vi "Keithley DMM7510 Acquire Triggered Multiple.vi"() -> ()   [LabVIEW 2015]
doc: "This example shows how to configure a measurement, set up triggering, trigger a measurement, and retrieve a measurement. It shows how to use the low-level Data VIs to retrieve data from the DMM."
uses:
  Keithley DMM7510.lvlib
panel:
  in  "Function":u16(ring) items=["Voltage: DC", "Voltage: AC", "Current: DC", "Current: AC", "2W Resistance", "4W Resistance", "Diode", "Capacitance", "Temperature", "Continuity", "Frequency", "Period", "Ratio"]
  in  "Sample Count (10)":i32=10 format="%#.6g"
  in  "Timeout (10000 ms)":i32=10000 format="%#.6g"
  out "Waveform Chart":dbl[](graph)
  in  "VISA resource name":refnum<visa-resource-name>
  # "(c) 2015 Keithley Instruments,,  ALL RIGHTS RESERVED."
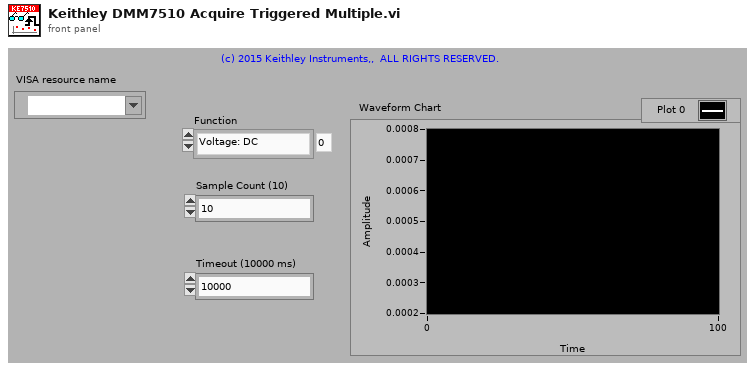
[diagram p1: front panel]
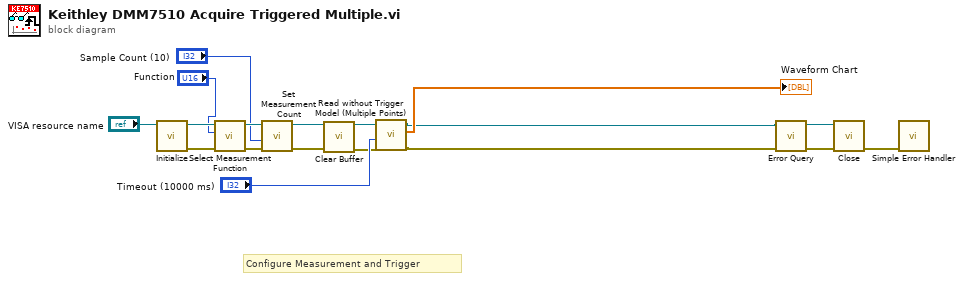
[diagram p0: block diagram]
diagram:
  # "Configure Measurement and Trigger"
  n1 = call "Initialize.vi"("VISA resource name"="VISA resource name") -> ("error out"=w14:errorcluster, "VISA resource name out"=w13:refnum<visa-resource-name>)  [unwired: 9 in]
  n2 = call "Select Measurement Function.vi"("error in (no error)"=w14, "Function"="Function", "VISA resource name"=w13) -> ("error out"=w11:errorcluster, "VISA resource name out"=w10:refnum<visa-resource-name>)  [unwired: 7 in]
  n3 = call "Set Measurement Count.vi"("error in (no error)"=w11, "Count"="Sample Count (10)", "VISA resource name"=w10) -> ("error out"=w4:errorcluster, "VISA resource name out"=w3:refnum<visa-resource-name>)  [unwired: 7 in]
  n4 = call "Clear Buffer.vi"("VISA resource name"=w3, "error in (no error)"=w4) -> ("VISA resource name out"=w2:refnum<visa-resource-name>, "error out"=w1:errorcluster)  [unwired: 12 in]
  n5 = call "Read without Trigger Model (Multiple Points).vi"("error in (no error)"=w1, "Timeout (10000 ms)"="Timeout (10000 ms)", "VISA resource name"=w2) -> ("error out"=w5:errorcluster, "Measurements"=→"Waveform Chart":dbl[], "VISA resource name out"=w6:refnum<visa-resource-name>)  [unwired: 5 in, 1 out]
  n6 = call "Error Query.vi"("error in (no error)"=w5, "VISA resource name"=w6) -> ("error out"=w15:errorcluster, "VISA resource name out"=w16:refnum<visa-resource-name>)  [unwired: 6 in, 2 out]
  n7 = call "Close.vi"("error in (no error)"=w15, "VISA resource name"=w16) -> ("error out"=w17:errorcluster)  [unwired: 9 in]
  n8 = call <vilib>:"Simple Error Handler.vi"("error in (no error)"=w17) -> ()  [unwired: 4 in, 5 out]
